vi "FBKdisplay.vi"() -> ()   [LabVIEW 2017]
uses:
  <vilib>/picture/3D Picture Control/NI_3D Picture Control.lvlib
  <vilib>/Utility/miscctls.llb/LVRectTypeDef.ctl
  <vilib>/picture/3D Picture Control/Object/Create Object (name).vi
panel:
  out "x-y":dbl
  out "ForceControl":bool
  out "HorizontalVisualFBK":bool
  out "InvertVisualFbk":bool
  in  "Render Dest":enum16{"Scene Window", "Scene Display"}(ring)
  in  "stop":bool
  in  "Camera Controller":enum16{"None", "Spherical", "Flying"}(ring)=enum."Spherical"
  out "error out":errorcluster
  out "Scene Display":refnum<vi>(3d-picture)
  out "error out 2":errorcluster
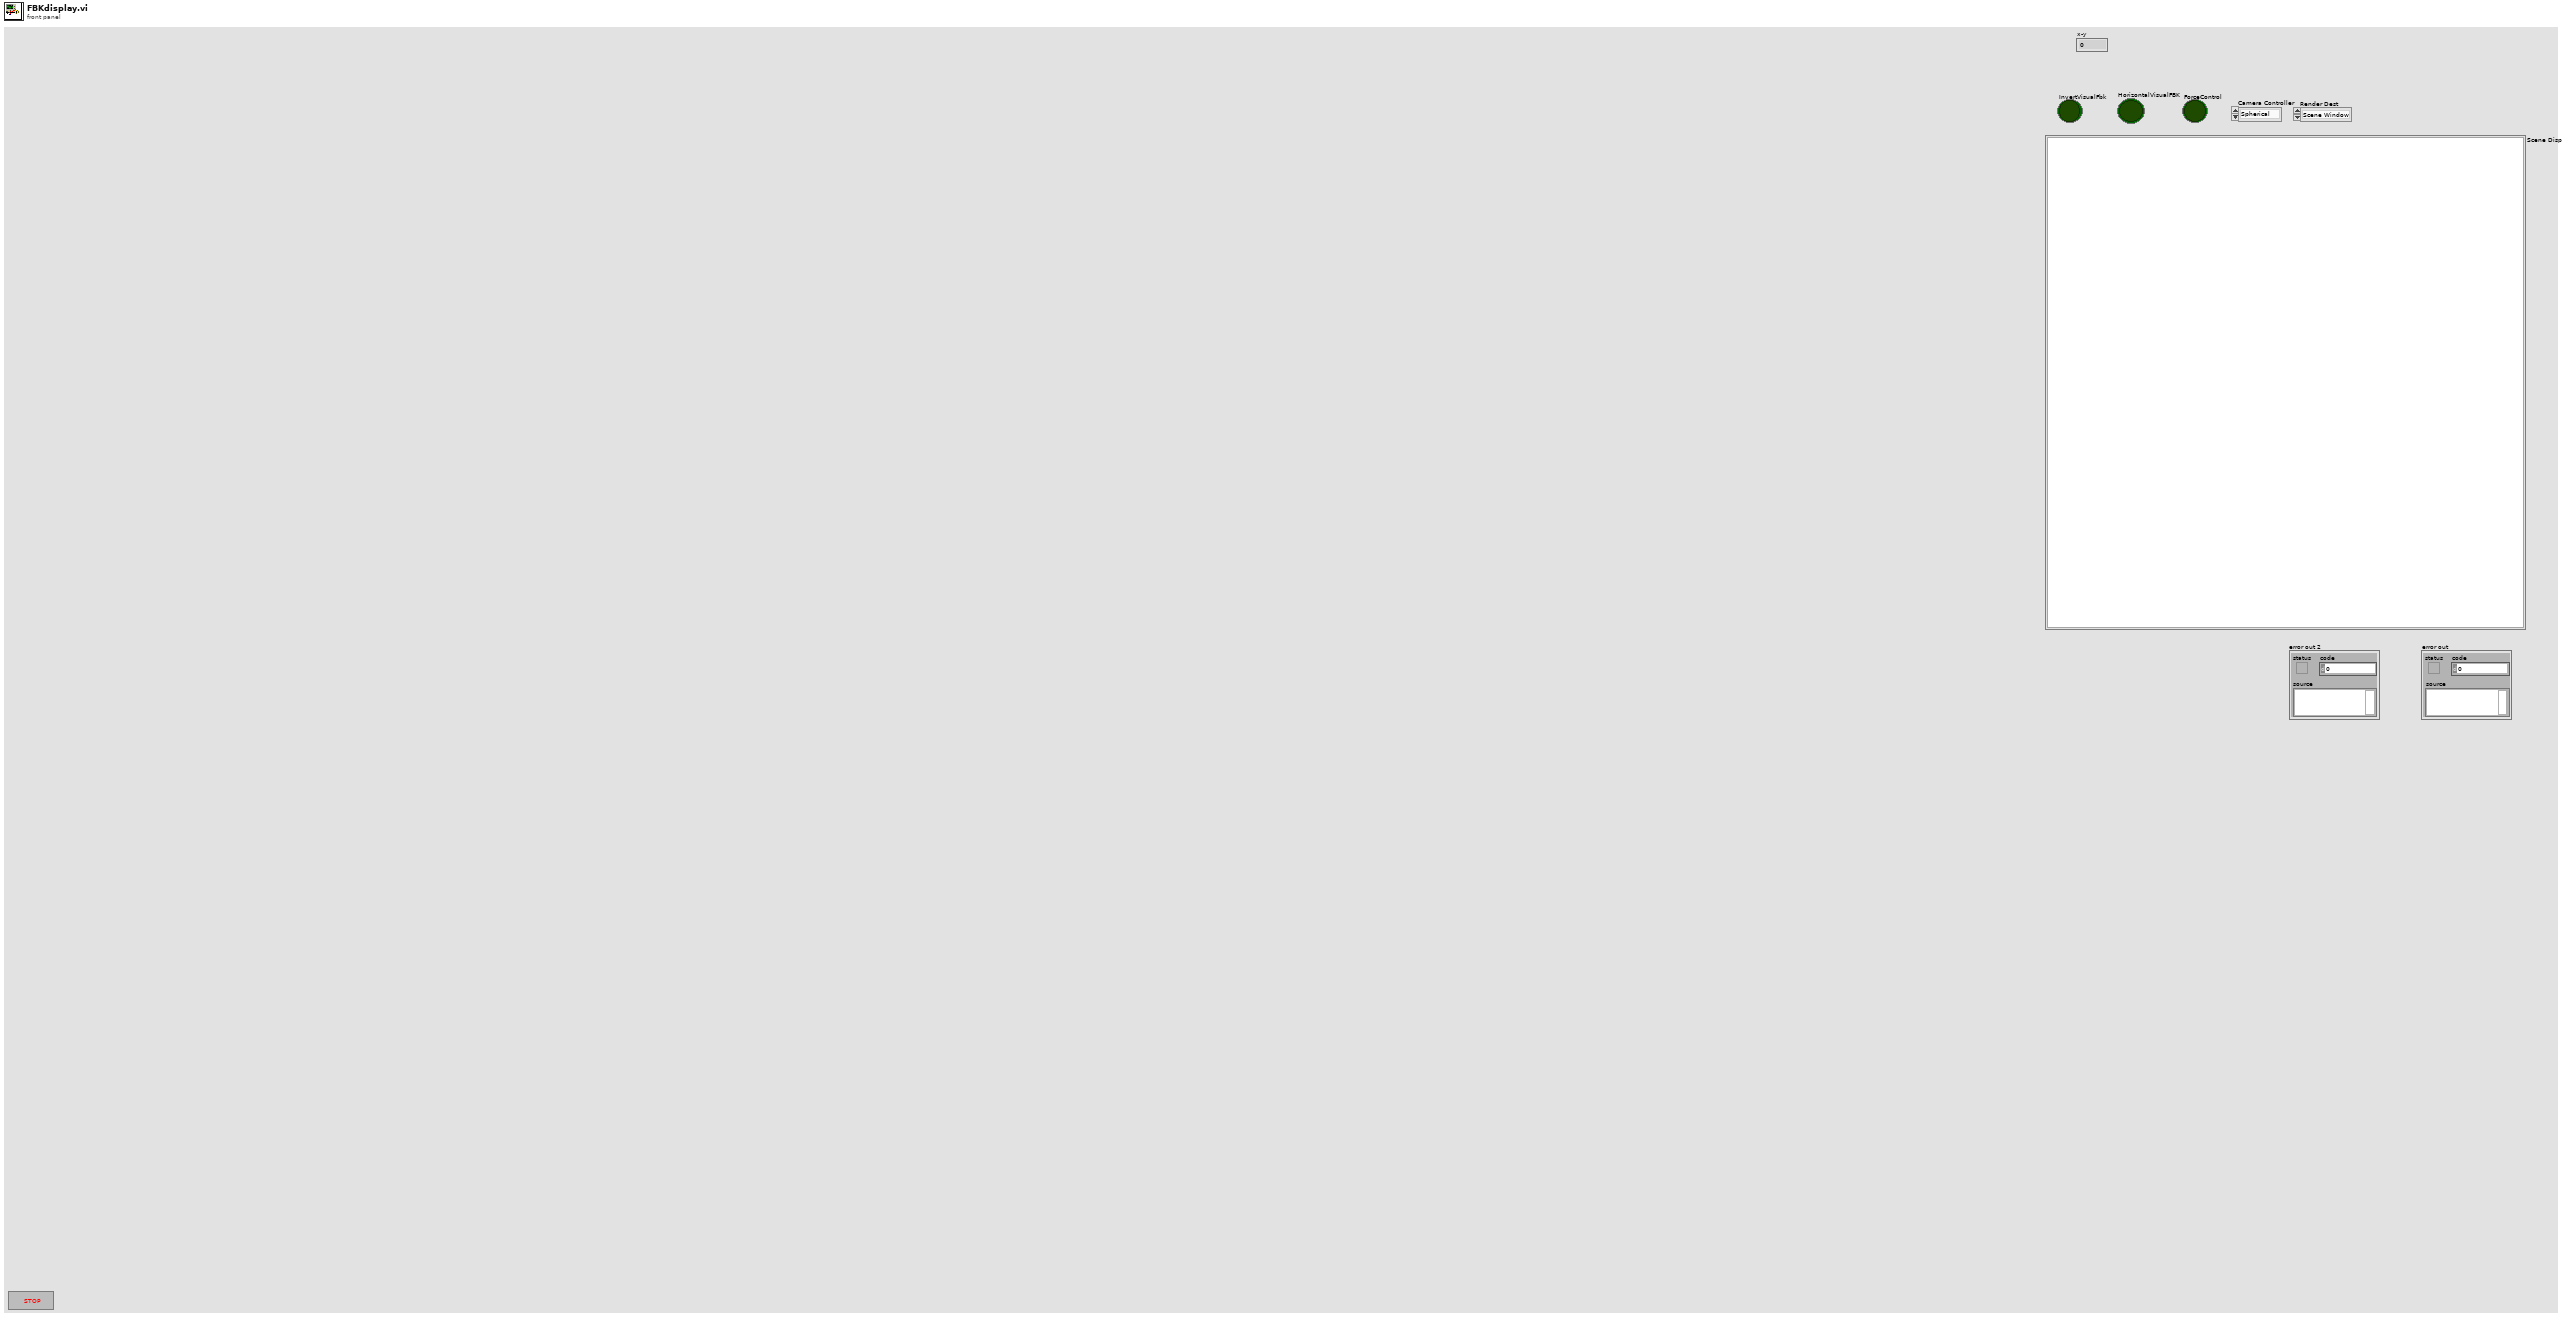
[diagram p1: front panel]
types:
  T1 = enum16{"As a Decal", "With Modulation", "With Blending", "As a replacement"}
  T2 = typedef "LVRectTypeDef.ctl" = cluster{"Left":i16, "Top":i16, "Right":i16, "Bottom":i16}
  T3 = enum16{"Open", "Minimized", "Maximized", "Hidden"}
  T4 = typedef "imagedata.ctl" = cluster{"image type":i32, "image depth":i32, "image":u8[], "mask":u8[], "colors":u32[], "Rectangle":cluster{"left":i16, "top":i16, "right":i16, "bottom":i16}}
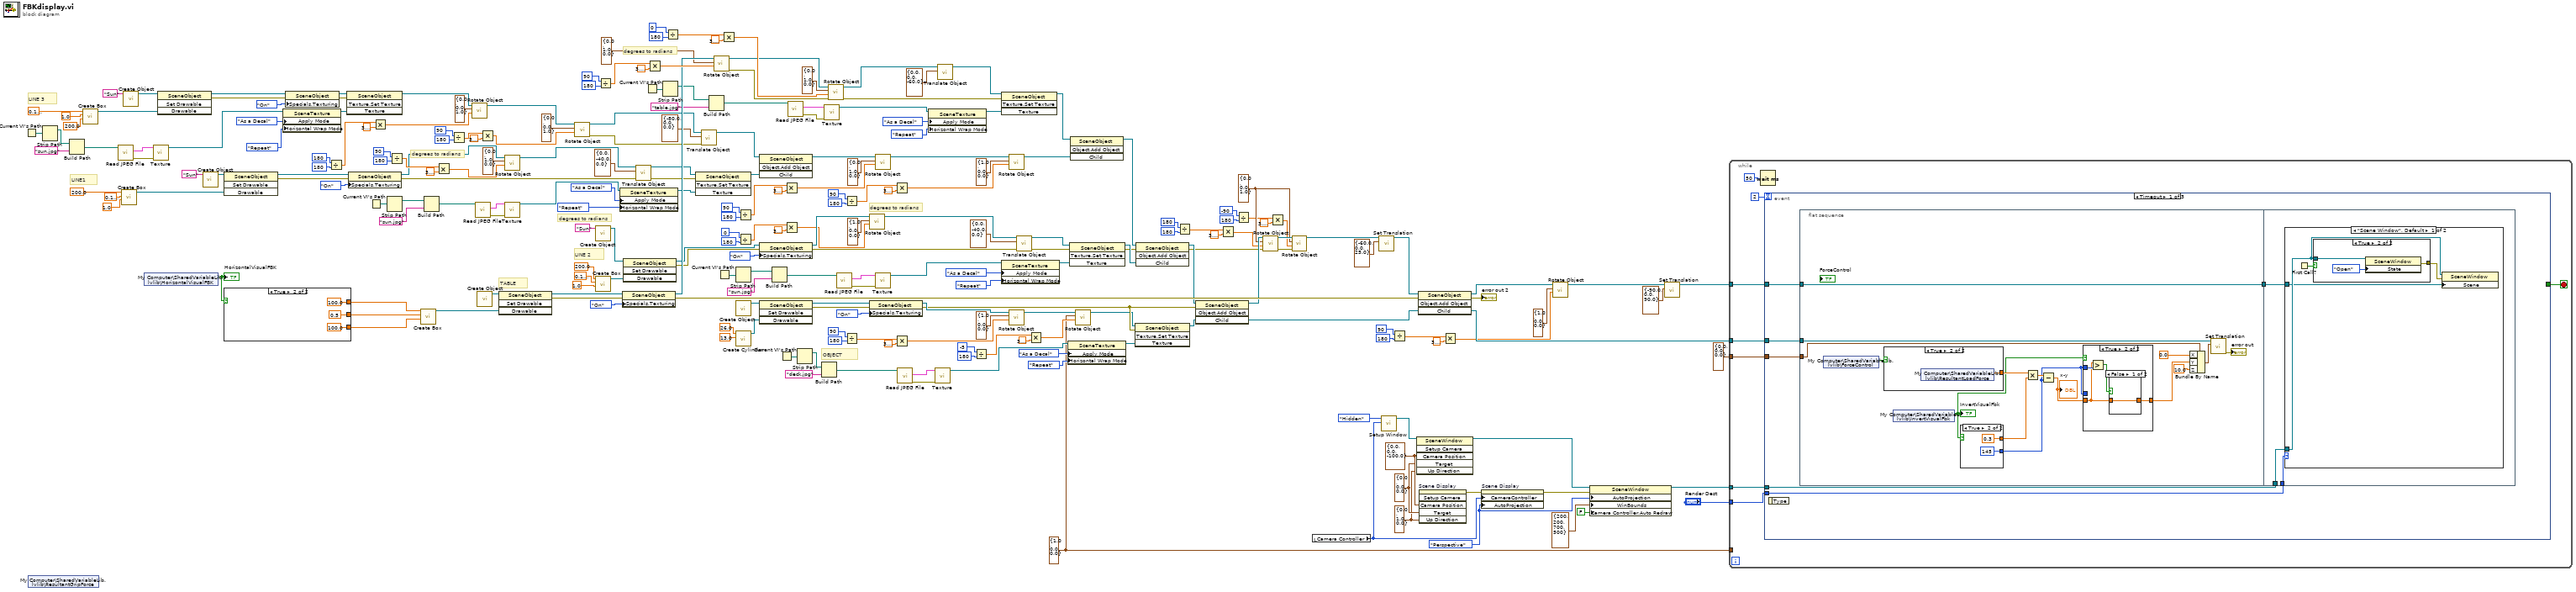
[diagram p0: block diagram]
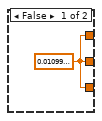
[diagram p2: hidden frame]
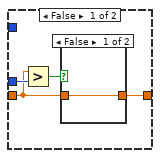
[diagram p3: hidden frame]
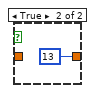
[diagram p4: hidden frame]
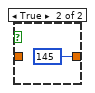
[diagram p5: hidden frame]
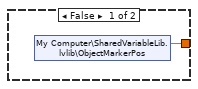
[diagram p6: hidden frame]
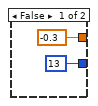
[diagram p7: hidden frame]
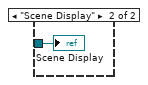
[diagram p9: hidden frame]
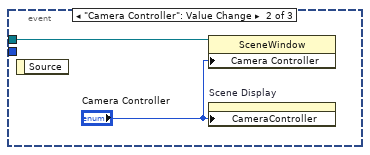
[diagram p10: hidden frame]
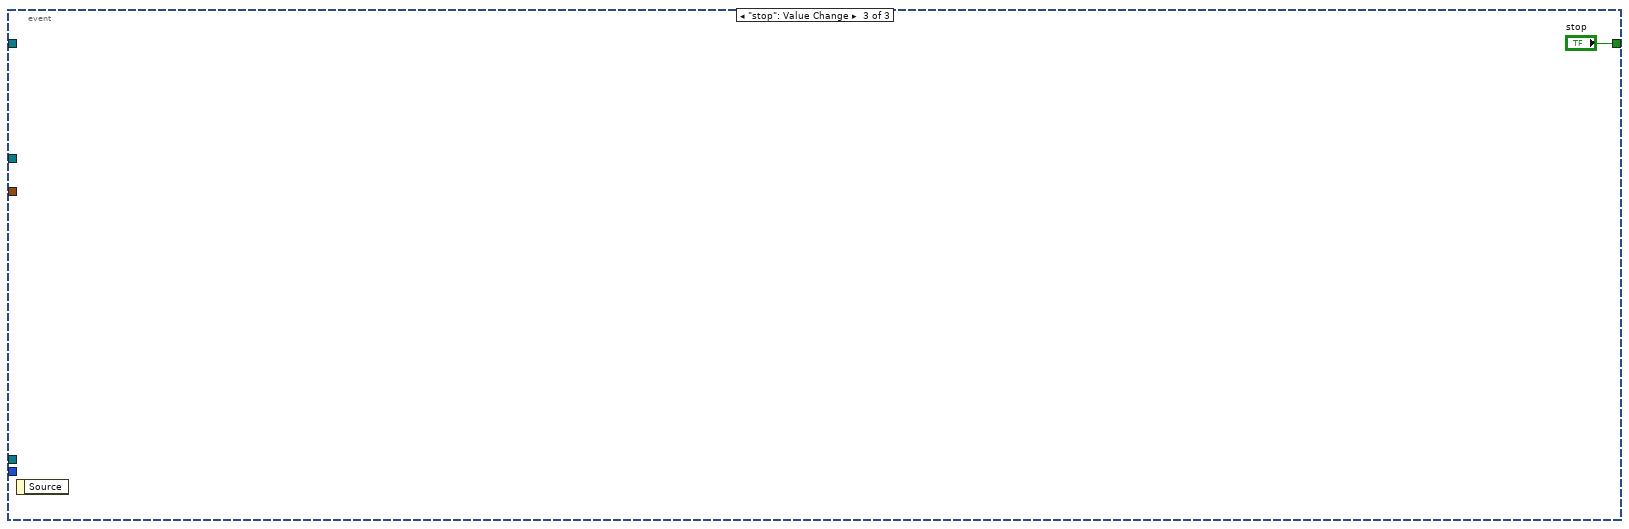
[diagram p11: hidden frame]
diagram:
  w74 = cluster{"X":sgl, "Y":sgl, "Z":sgl} {"X"=0.0, "Y"=0.0, "Z"=1.0} ("Axis")
  w119 = cluster{"X":sgl, "Y":sgl, "Z":sgl} {"X"=1.0, "Y"=0.0, "Z"=0.0} ("Axis")
  w212 = enum16{"None", "Perspective", "Orthographic"}."Perspective" ("Auto Projection Mode")
  w215 = cluster{"X":sgl, "Y":sgl, "Z":sgl} {"X"=0.0, "Y"=1.0, "Z"=0.0} ("Up Direction")
  w216 = cluster{"X":sgl, "Y":sgl, "Z":sgl} {"X"=0.0, "Y"=0.0, "Z"=0.0} ("Target")
  w217 = cluster{"X":sgl, "Y":sgl, "Z":sgl} {"X"=0.0, "Y"=0.0, "Z"=-100.0} ("Camera Position")
  # "degrees to radians"
  # "LINE 3"
  # "OBJECT"
  # "LINE 2"
  # "LINE1"
  # "TABLE"
  # "degrees to radians"
  # "degrees to radians"
  # "degrees to radians"
  n1 = Current VI's Path() -> (path=w110:path)
  n2 = shared-variable "My Computer\\SharedVariableLib.lvlib\\ResultantGripForce"() -> ()  [unwired: 1 in, 2 out]
  n3 = Strip Path(path=w110) -> (stripped path=w109:path)  [unwired: 1 out]
  n4 = Build Path(base path=w109, name or relative path="sun.jpg" ("Name")) -> (appended path=w107:path)
  n5 = call <vilib>:"Create Box.vi"("Length Z"=sgl 200.0 ("Detail"), "Length Y"=sgl 1.0 ("Detail"), "Length X"=sgl 0.1 ("Radius")) -> ("New Box Refnum"=w116:refnum<vi>)  [unwired: 7 in, 1 out]
  n6 = call <vilib>:"Read JPEG File.vi"("path to JPEG file"=w107) -> ("error out"=w111:errorcluster, "image data"=w112:T4)  [unwired: 1 in, 8 out]
  n7 = call <vilib>:"Create Box.vi"("Length Z"=sgl 1.0 ("Detail"), "Length Y"=sgl 0.1 ("Detail"), "Length X"=sgl 200.0 ("Radius")) -> ("New Box Refnum"=w179:refnum<vi>)  [unwired: 7 in, 1 out]
  n8 = call-poly <vilib>:"Create Object.vi"("Name"="Sun") -> ("Scene:New Object"=w117:refnum<vi>)  [unwired: 9 in, 1 out]
  n9 = shared-variable "My Computer\\SharedVariableLib.lvlib\\HorizontalVisualFBK"() -> (w4:bool)  [unwired: 1 in, 1 out]
  "HorizontalVisualFBK" <- w4
  n10 = call <vilib>:"Texture.vi"("error in (no error)"=w111, "Image"=w112) -> ("New Texture Refnum"=w102:refnum<vi>)  [unwired: 9 out]
  n11 = invoke class="SceneObject" method="Set Drawable"(reference=w117, "Drawable"=w116) -> (reference out=w106:refnum<vi>, error out=w105:errorcluster)  [unwired: 2 in, 2 out]
  n12 = call-poly <vilib>:"Create Object.vi"("Name"="Sun") -> ("Scene:New Object"=w180:refnum<vi>)  [unwired: 9 in, 1 out]
  n13 = invoke class="SceneObject" method="Set Drawable"(reference=w180, "Drawable"=w179) -> (reference out=w177:refnum<vi>, error out=w176:errorcluster)  [unwired: 2 in, 2 out]
  n14 = case shown="True" w4 {
    tunnel: [w242 sgl 100.0 ("Radius")] -> w1
    tunnel: [w242 sgl 0.5 ("Radius")] -> w2
    tunnel: [w242 sgl 100.0 ("Radius")] -> w3
    frame False {
      w242 = sgl 0.011 ("Radius")
    }
    frame True {
    }
  }
  n15 = property class="SceneTexture"(reference=w102, "Apply Mode"=T1."As a Decal", "Horizontal Wrap Mode"=enum16{"Clamp", "Repeat"}."Repeat") -> (reference out=w100:refnum<vi>)  [unwired: 1 in, 1 out]
  n16 = property class="SceneObject"(reference=w106, error in=w105, "Specials.Texturing"=enum16{"Inherit Value", "Off", "On"}."On" ("Specials:Texturing")) -> (reference out=w11:refnum<vi>, error out=w10:errorcluster)
  n17 = Divide(x=180, y=180) -> (x/y=w39:dbl)
  n18 = invoke class="SceneObject" method="Texture.Set Texture"(reference=w11, error in=w10, "Texture"=w100) -> (reference out=w44:refnum<vi>)  [unwired: 1 in, 3 out]
  n19 = property class="SceneObject"(reference=w177, error in=w176, "Specials.Texturing"=enum16{"Inherit Value", "Off", "On"}."On" ("Specials:Texturing")) -> (reference out=w159:refnum<vi>, error out=w129:errorcluster)
  n20 = Current VI's Path() -> (path=w169:path)
  n21 = Multiply(x=w39, y=3.141592653589793) -> (x*y=w38:dbl)
  n22 = Strip Path(path=w169) -> (stripped path=w168:path)  [unwired: 1 out]
  n23 = Divide(x=90, y=180) -> (x/y=w160:dbl)
  n24 = call <vilib>:"Create Box.vi"("Length Z"=w1, "Length Y"=w2, "Length X"=w3) -> ("New Box Refnum"=w221:refnum<vi>)  [unwired: 7 in, 1 out]
  n25 = Build Path(base path=w168, name or relative path="sun.jpg" ("Name")) -> (appended path=w166:path)
  n26 = Multiply(x=w160, y=3.141592653589793) -> (x*y=w61:dbl)
  n27 = Divide(x=90, y=180) -> (x/y=w32:dbl)
  n28 = call <vilib>:"Rotate Object.vi"("Angle"=w38, "Axis"=cluster{"X":sgl, "Y":sgl, "Z":sgl} {"X"=0.0, "Y"=0.0, "Z"=1.0}, "Scene.Object In"=w44) -> ("Scene.Object Out"=w36:refnum<vi>)  [unwired: 1 in, 7 out]
  n29 = call <vilib>:"Read JPEG File.vi"("path to JPEG file"=w166) -> ("error out"=w171:errorcluster, "image data"=w172:T4)  [unwired: 1 in, 8 out]
  n30 = call-poly <vilib>:"Create Object.vi"() -> ("Scene:New Object"=w229:refnum<vi>)  [unwired: 10 in, 1 out]
  n31 = Multiply(x=w32, y=3.141592653589793) -> (x*y=w31:dbl)
  n32 = invoke class="SceneObject" method="Set Drawable"(reference=w229, "Drawable"=w221) -> (reference out=w241:refnum<vi>, error out=w240:errorcluster)  [unwired: 2 in, 2 out]
  n33 = call <vilib>:"Texture.vi"("error in (no error)"=w171, "Image"=w172) -> ("New Texture Refnum"=w170:refnum<vi>)  [unwired: 9 out]
  n34 = call <vilib>:"Rotate Object.vi"("Angle"=w61, "Axis"=cluster{"X":sgl, "Y":sgl, "Z":sgl} {"X"=0.0, "Y"=1.0, "Z"=0.0}, "Scene.Object In"=w159) -> ("Scene.Object Out"=w45:refnum<vi>)  [unwired: 1 in, 7 out]
  n35 = call <vilib>:"Rotate Object.vi"("Angle"=w31, "Axis"=cluster{"X":sgl, "Y":sgl, "Z":sgl} {"X"=0.0, "Y"=0.0, "Z"=1.0}, "Scene.Object In"=w36) -> ("error out"=w28:errorcluster, "Scene.Object Out"=w29:refnum<vi>)  [unwired: 1 in, 6 out]
  n36 = call-poly <vilib>:"Create Object.vi"("Name"="Sun") -> ("Scene:New Object"=w157:refnum<vi>)  [unwired: 9 in, 1 out]
  n37 = call <vilib>:"Create Box.vi"("Length Z"=sgl 1.0 ("Detail"), "Length Y"=sgl 0.1 ("Detail"), "Length X"=sgl 200.0 ("Radius")) -> ("New Box Refnum"=w156:refnum<vi>)  [unwired: 7 in, 1 out]
  n38 = Divide(x=90, y=180) -> (x/y=w235:dbl)
  n39 = property class="SceneTexture"(reference=w170, "Apply Mode"=T1."As a Decal", "Horizontal Wrap Mode"=enum16{"Clamp", "Repeat"}."Repeat") -> (reference out=w99:refnum<vi>)  [unwired: 1 in, 1 out]
  n40 = property class="SceneObject"(reference=w241, error in=w240, "Specials.Texturing"=enum16{"Inherit Value", "Off", "On"}."On" ("Specials:Texturing")) -> (reference out=w225:refnum<vi>, error out=w134:errorcluster)
  n41 = invoke class="SceneObject" method="Set Drawable"(reference=w157, "Drawable"=w156) -> (reference out=w154:refnum<vi>, error out=w153:errorcluster)  [unwired: 2 in, 2 out]
  n42 = call <vilib>:"Translate Object.vi"("error in (no error)"=w129, "Translation"=cluster{"X":sgl, "Y":sgl, "Z":sgl} {"X"=0.0, "Y"=-40.0, "Z"=0.0} ("Axis"), "Scene.Object In"=w45) -> ("error out"=w97:errorcluster, "Scene.Object Out"=w98:refnum<vi>)  [unwired: 7 in]
  n43 = Current VI's Path() -> (path=w194:path)
  n44 = Multiply(x=w235, y=3.141592653589793) -> (x*y=w227:dbl)
  n45 = Strip Path(path=w194) -> (stripped path=w193:path)  [unwired: 1 out]
  n46 = Divide(x=0, y=180) -> (x/y=w200:dbl)
  n47 = invoke class="SceneObject" method="Texture.Set Texture"(reference=w98, error in=w97, "Texture"=w99) -> (reference out=w96:refnum<vi>)  [unwired: 1 in, 3 out]
  n48 = call <vilib>:"Translate Object.vi"("error in (no error)"=w28, "Translation"=cluster{"X":sgl, "Y":sgl, "Z":sgl} {"X"=-80.0, "Y"=0.0, "Z"=0.0} ("Axis"), "Scene.Object In"=w29) -> ("Scene.Object Out"=w27:refnum<vi>)  [unwired: 7 in, 1 out]
  n49 = Build Path(base path=w193, name or relative path="table.jpg" ("Name")) -> (appended path=w191:path)
  n50 = call <vilib>:"Rotate Object.vi"("Angle"=w227, "Axis"=cluster{"X":sgl, "Y":sgl, "Z":sgl} {"X"=0.0, "Y"=1.0, "Z"=0.0}, "Scene.Object In"=w225) -> ("error out"=w198:errorcluster, "Scene.Object Out"=w197:refnum<vi>)  [unwired: 1 in, 6 out]
  n51 = Current VI's Path() -> (path=w146:path)
  n52 = Multiply(x=w200, y=3.141592653589793) -> (x*y=w199:dbl)
  n53 = Strip Path(path=w146) -> (stripped path=w145:path)  [unwired: 1 out]
  n54 = call-poly <vilib>:"Create Object.vi"() -> ("Scene:New Object"=w228:refnum<vi>)  [unwired: 10 in, 1 out]
  n55 = call <vilib>:"Create Cylinder.vi"("Radius"=sgl 13.0 ("Detail"), "Height"=sgl 26.0 ("Radius")) -> ("New Cylinder Refnum"=w220:refnum<vi>)  [unwired: 8 in, 1 out]
  n56 = Divide(x=90, y=180) -> (x/y=w65:dbl)
  n57 = Divide(x=0, y=180) -> (x/y=w137:dbl)
  n58 = invoke class="SceneObject" method="Object.Add Object"(reference=w27, "Child"=w96) -> (reference out=w48:refnum<vi>)  [unwired: 2 in, 3 out]
  n59 = property class="SceneObject"(reference=w154, error in=w153, "Specials.Texturing"=enum16{"Inherit Value", "Off", "On"}."On" ("Specials:Texturing")) -> (reference out=w136:refnum<vi>, error out=w93:errorcluster)
  n60 = invoke class="SceneObject" method="Set Drawable"(reference=w228, "Drawable"=w220) -> (reference out=w231:refnum<vi>, error out=w233:errorcluster)  [unwired: 2 in, 2 out]
  n61 = Build Path(base path=w145, name or relative path="sun.jpg" ("Name")) -> (appended path=w143:path)
  n62 = Current VI's Path() -> (path=w187:path)
  n63 = Multiply(x=w65, y=3.141592653589793) -> (x*y=w63:dbl)
  n64 = Multiply(x=w137, y=3.141592653589793) -> (x*y=w59:dbl)
  n65 = call <vilib>:"Read JPEG File.vi"("path to JPEG file"=w191) -> ("error out"=w195:errorcluster, "image data"=w196:T4)  [unwired: 1 in, 8 out]
  n66 = Strip Path(path=w187) -> (stripped path=w186:path)  [unwired: 1 out]
  n67 = Build Path(base path=w186, name or relative path="deck.jpg" ("Name")) -> (appended path=w184:path)
  n68 = call <vilib>:"Texture.vi"("error in (no error)"=w195, "Image"=w196) -> ("New Texture Refnum"=w88:refnum<vi>)  [unwired: 9 out]
  n69 = call <vilib>:"Rotate Object.vi"("error in (no error)"=w198, "Angle"=w199, "Axis"=cluster{"X":sgl, "Y":sgl, "Z":sgl} {"X"=0.0, "Y"=1.0, "Z"=0.0}, "Scene.Object In"=w197) -> ("error out"=w9:errorcluster, "Scene.Object Out"=w7:refnum<vi>)  [unwired: 6 out]
  n70 = call <vilib>:"Read JPEG File.vi"("path to JPEG file"=w143) -> ("error out"=w148:errorcluster, "image data"=w149:T4)  [unwired: 1 in, 8 out]
  n71 = Divide(x=90, y=180) -> (x/y=w55:dbl)
  n72 = Divide(x=90, y=180) -> (x/y=w128:dbl)
  n73 = call <vilib>:"Rotate Object.vi"("Angle"=w59, "Axis"=cluster{"X":sgl, "Y":sgl, "Z":sgl} {"X"=1.0, "Y"=0.0, "Z"=0.0}, "Scene.Object In"=w136) -> ("Scene.Object Out"=w49:refnum<vi>)  [unwired: 1 in, 7 out]
  n74 = property class="SceneObject"(reference=w231, error in=w233, "Specials.Texturing"=enum16{"Inherit Value", "Off", "On"}."On" ("Specials:Texturing")) -> (reference out=w121:refnum<vi>, error out=w15:errorcluster)
  n75 = call <vilib>:"Texture.vi"("error in (no error)"=w148, "Image"=w149) -> ("New Texture Refnum"=w147:refnum<vi>)  [unwired: 9 out]
  n76 = call <vilib>:"Rotate Object.vi"("Angle"=w63, "Axis"=cluster{"X":sgl, "Y":sgl, "Z":sgl} {"X"=0.0, "Y"=1.0, "Z"=0.0}, "Scene.Object In"=w48) -> ("Scene.Object Out"=w52:refnum<vi>)  [unwired: 1 in, 7 out]
  n77 = Multiply(x=w55, y=3.141592653589793) -> (x*y=w54:dbl)
  n78 = Multiply(x=w128, y=3.141592653589793) -> (x*y=w222:dbl)
  n79 = call <vilib>:"Read JPEG File.vi"("path to JPEG file"=w184) -> ("error out"=w189:errorcluster, "image data"=w190:T4)  [unwired: 1 in, 8 out]
  n80 = property class="SceneTexture"(reference=w88, "Apply Mode"=T1."As a Decal", "Horizontal Wrap Mode"=enum16{"Clamp", "Repeat"}."Repeat") -> (reference out=w87:refnum<vi>)  [unwired: 1 in, 1 out]
  n81 = call <vilib>:"Texture.vi"("error in (no error)"=w189, "Image"=w190) -> ("New Texture Refnum"=w188:refnum<vi>)  [unwired: 9 out]
  n82 = call <vilib>:"Translate Object.vi"("Translation"=cluster{"X":sgl, "Y":sgl, "Z":sgl} {"X"=0.0, "Y"=0.0, "Z"=-60.0}, "Scene.Object In"=w7) -> ("Scene.Object Out"=w6:refnum<vi>)  [unwired: 8 in, 1 out]
  n83 = Divide(x=-5, y=180) -> (x/y=w123:dbl)
  n84 = property class="SceneTexture"(reference=w147, "Apply Mode"=T1."As a Decal", "Horizontal Wrap Mode"=enum16{"Clamp", "Repeat"}."Repeat") -> (reference out=w92:refnum<vi>)  [unwired: 1 in, 1 out]
  n85 = invoke class="SceneObject" method="Texture.Set Texture"(reference=w6, error in=w9, "Texture"=w87) -> (reference out=w84:refnum<vi>)  [unwired: 1 in, 3 out]
  n86 = call <vilib>:"Rotate Object.vi"("Angle"=w54, "Axis"=cluster{"X":sgl, "Y":sgl, "Z":sgl} {"X"=1.0, "Y"=0.0, "Z"=0.0}, "Scene.Object In"=w52) -> ("Scene.Object Out"=w51:refnum<vi>)  [unwired: 1 in, 7 out]
  n87 = call <vilib>:"Rotate Object.vi"("Angle"=w222, "Axis"=cluster{"X":sgl, "Y":sgl, "Z":sgl} {"X"=1.0, "Y"=0.0, "Z"=0.0}, "Scene.Object In"=w121) -> ("Scene.Object Out"=w120:refnum<vi>)  [unwired: 1 in, 7 out]
  n88 = call <vilib>:"Translate Object.vi"("error in (no error)"=w93, "Translation"=cluster{"X":sgl, "Y":sgl, "Z":sgl} {"X"=0.0, "Y"=-40.0, "Z"=0.0} ("Axis"), "Scene.Object In"=w49) -> ("error out"=w94:errorcluster, "Scene.Object Out"=w95:refnum<vi>)  [unwired: 7 in]
  n89 = Multiply(x=w123, y=3.141592653589793) -> (x*y=w125:dbl)
  n90 = property class="SceneTexture"(reference=w188, "Apply Mode"=T1."As a Decal", "Horizontal Wrap Mode"=enum16{"Clamp", "Repeat"}."Repeat") -> (reference out=w133:refnum<vi>)  [unwired: 1 in, 1 out]
  n91 = invoke class="SceneObject" method="Texture.Set Texture"(reference=w95, error in=w94, "Texture"=w92) -> (reference out=w91:refnum<vi>, error out=w14:errorcluster)  [unwired: 1 in, 2 out]
  n92 = invoke class="SceneObject" method="Object.Add Object"(reference=w84, "Child"=w51) -> (reference out=w47:refnum<vi>)  [unwired: 2 in, 3 out]
  n93 = call <vilib>:"Rotate Object.vi"("Angle"=w125, "Axis"=w119, "Scene.Object In"=w120) -> ("Scene.Object Out"=w8:refnum<vi>)  [unwired: 1 in, 7 out]
  n94 = invoke class="SceneObject" method="Texture.Set Texture"(reference=w8, error in=w15, "Texture"=w133) -> (reference out=w132:refnum<vi>)  [unwired: 1 in, 3 out]
  n95 = invoke class="SceneObject" method="Object.Add Object"(reference=w47, error in=w14, "Child"=w91) -> (reference out=w46:refnum<vi>, error out=w13:errorcluster)  [unwired: 1 in, 2 out]
  n96 = Divide(x=180, y=180) -> (x/y=w80:dbl)
  n97 = invoke class="SceneObject" method="Object.Add Object"(reference=w46, error in=w15, "Child"=w132) -> (reference out=w83:refnum<vi>, "Child"=w26:refnum<vi>)  [unwired: 1 in, 2 out]
  n98 = Multiply(x=w80, y=3.141592653589793) -> (x*y=w78:dbl)
  n99 = Divide(x=-90, y=180) -> (x/y=w71:dbl)
  n100 = call <vilib>:"Rotate Object.vi"("error in (no error)"=w13, "Angle"=w78, "Axis"=w74, "Scene.Object In"=w83) -> ("error out"=w12:errorcluster, "Scene.Object Out"=w75:refnum<vi>)  [unwired: 6 out]
  n101 = Multiply(x=w71, y=3.141592653589793) -> (x*y=w69:dbl)
  n102 = call <vilib>:"Rotate Object.vi"("error in (no error)"=w12, "Angle"=w69, "Axis"=w74, "Scene.Object In"=w75) -> ("Scene.Object Out"=w68:refnum<vi>)  [unwired: 7 out]
  n103 = local read "Camera Controller"() -> (w209:enum16{"None", "Spherical", "Flying"})
  n104 = call <vilib>:"Set Translation.vi"("Translation"=cluster{"X":sgl, "Y":sgl, "Z":sgl} {"X"=-60.0, "Y"=0.0, "Z"=25.0}, "Scene Object"=w68) -> ("Translated Object"=w77:refnum<vi>)  [unwired: 8 in, 1 out]
  n105 = call <vilib>:"Setup Window.vi"("Camera Controller"=w209, "Window State"=T3."Hidden") -> ("New Window Refnum"=w211:refnum<vi>)  [unwired: 1 in, 8 out]
  n106 = Divide(x=90, y=180) -> (x/y=w22:dbl)
  n107 = invoke class="SceneWindow" method="Setup Camera"(reference=w211, "Camera Position"=w217, "Target"=w216, "Up Direction"=w215) -> (reference out=w218:refnum<vi>)  [unwired: 2 in, 5 out]
  n108 = invoke class="SceneObject" method="Object.Add Object"(reference=w77, error in=w134, "Child"=w26) -> (reference out=w18:refnum<vi>, error out=→"error out 2":errorcluster, "Child"=w131:refnum<vi>)  [unwired: 1 in, 1 out]
  n109 = invoke on="Scene Display" class="SceneGraphDisp (strict)" method="Setup Camera"("Camera Position"=w217, "Target"=w216, "Up Direction"=w215) -> (error out=w214:errorcluster)  [unwired: 3 in, 5 out]
  n110 = Multiply(x=w22, y=3.141592653589793) -> (x*y=w20:dbl)
  n111 = property on="Scene Display" class="SceneGraphDisp (strict)"(error in=w214, "CameraController"=w209, "AutoProjection"=w212) -> (error out=w213:errorcluster)  [unwired: 1 in, 1 out]
  n112 = call <vilib>:"Rotate Object.vi"("Angle"=w20, "Axis"=cluster{"X":sgl, "Y":sgl, "Z":sgl} {"X"=1.0, "Y"=0.0, "Z"=0.0}, "Scene.Object In"=w18) -> ("Scene.Object Out"=w17:refnum<vi>)  [unwired: 1 in, 7 out]
  n113 = property class="SceneWindow"(reference=w218, error in=w213, "AutoProjection"=w212, "WinBounds"=T2 {"Left"=200, "Top"=200, "Right"=700, "Bottom"=500} ("Window Bounds"), "Camera Controller.Auto Redraw"=FALSE ("Camera Controller:Auto Redraw")) -> (reference out=w205:refnum<vi>)  [unwired: 1 out]
  n114 = call <vilib>:"Set Translation.vi"("Translation"=cluster{"X":sgl, "Y":sgl, "Z":sgl} {"X"=-90.0, "Y"=0.0, "Z"=90.0}, "Scene Object"=w17) -> ("Translated Object"=w16:refnum<vi>)  [unwired: 8 in, 1 out]
  n115 = while {
    tunnel: w131 -> [w250]
    tunnel: w16 -> [w251]
    tunnel: "Render Dest" -> [w247]
    tunnel: w205 -> [w249]
    tunnel: cluster{"X":sgl, "Y":sgl, "Z":sgl} {"X"=0.0, "Y"=0.0, "Z"=0.0} ("Translation") -> [w246]
    tunnel: w119 -> [_]
    stop <- w248 stop-if-true
    n116 = Wait (ms)(milliseconds to wait=u32 50) -> ()  [unwired: 1 out]
    n117 = event shown="[0] Timeout" {
      selector: _ -> [_ _ _]
      dyn-events: _ -> [_ _ _]
      timeout: 2 -> [_ _ _]
      tunnel: [_ _ "stop"] -> w248
      tunnel: w251 -> [w258 _ _]
      tunnel: w250 -> [w257 _ _]
      tunnel: w246 -> [w256 _ _]
      tunnel: w247 -> [w255 _ _]
      tunnel: w249 -> [w254 w305 _]
      event Timeout {
        n118 = event-data() -> ()  [unwired: 2 out]
        n119 = flat-sequence {
          tunnel: [w274] -> w259
          tunnel: w256 -> [w266]
          tunnel: w257 -> [w267]
          tunnel: w258 -> [w274]
          tunnel: w259 -> [w295]
          tunnel: w255 -> [w294]
          tunnel: w254 -> [w293]
          frame #0 {
            n120 = shared-variable "My Computer\\SharedVariableLib.lvlib\\ForceControl"() -> (w264:bool)  [unwired: 1 in, 1 out]
            n121 = case shown="True" w264 {
              tunnel: [w287 w288] -> w265
              frame False {
                n122 = shared-variable "My Computer\\SharedVariableLib.lvlib\\ObjectMarkerPos"() -> (w287:dbl)  [unwired: 1 in, 1 out]
              }
              frame True {
                n123 = shared-variable "My Computer\\SharedVariableLib.lvlib\\ResultantLoadForce"() -> (w288:dbl)  [unwired: 1 in, 1 out]
              }
            }
            n124 = shared-variable "My Computer\\SharedVariableLib.lvlib\\InvertVisualFbk"() -> (w263:bool)  [unwired: 1 in, 1 out]
            "InvertVisualFbk" <- w263
            n125 = case shown="True" w263 {
              tunnel: [13 145] -> w260
              tunnel: [-0.3 0.3] -> w268
              frame False {
              }
              frame True {
              }
            }
            n126 = Multiply(x=w265, y=w268) -> (x*y=w269:dbl)
            n127 = Subtract(x=w269, y=w260) -> (x-y=w262:dbl)
            "x-y" <- w262
            n128 = case shown="True" w263 {
              tunnel: w262 -> [w275 w281]
              tunnel: w260 -> [w278 _]
              tunnel: [w276 w282] -> w261
              tunnel: w260 -> [_ w283]
              frame False {
                n129 = Greater?(x=w275, y=w278) -> (0:w277:bool)
                n130 = case shown="False" w277 {
                  tunnel: [w279 13] -> w276
                  tunnel: w275 -> [w279 _]
                  frame False {
                  }
                  frame True {
                  }
                }
              }
              frame True {
                n131 = Greater?(x=w281, y=w283) -> (0:w284:bool)
                n132 = case shown="False" w284 {
                  tunnel: [w285 145] -> w282
                  tunnel: w281 -> [w285 _]
                  frame False {
                  }
                  frame True {
                  }
                }
              }
            }
            n133 = Bundle By Name(cluster=w266, "X"=sgl 0.0, "Y"=w261, "Z"=sgl 10.0) -> (w271:cluster{"X":sgl, "Y":sgl, "Z":sgl})
            n134 = call <vilib>:"Set Translation.vi"("Translation"=w271, "Scene Object"=w267) -> ("error out"=→"error out":errorcluster)  [unwired: 8 in, 1 out]
          }
          frame #1 {
            n135 = case shown="\"Scene Window\", Default" w294 {
              tunnel: w293 -> [w297 _]
              tunnel: w295 -> [w296 w303]
              frame "Scene Window", Default {
                n136 = First Call?() -> (First Call?: T/F=w298:bool)
                n137 = case shown="True" w298 {
                  tunnel: w297 -> [_ w302]
                  tunnel: [_ w301] -> w299
                  frame False {
                  }
                  frame True {
                    n138 = property class="SceneWindow"(reference=w302, "State"=T3."Open" ("Window State")) -> (error out=w301:errorcluster)  [unwired: 1 in, 1 out]
                  }
                }
                n139 = property class="SceneWindow"(reference=w297, error in=w299, "Scene"=w296) -> ()  [unwired: 2 out]
              }
              frame "Scene Display" {
                "Scene Display" <- w303
              }
            }
          }
        }
      }
      event "Camera Controller": Value Change {
        n140 = event-data() -> ()  [unwired: 2 out]
        n141 = property class="SceneWindow"(reference=w305, "Camera Controller"="Camera Controller") -> ()  [unwired: 1 in, 2 out]
        n142 = property on="Scene Display" class="SceneGraphDisp (strict)"("CameraController"="Camera Controller") -> ()  [unwired: 2 in, 2 out]
      }
      event "stop": Value Change {
        n143 = event-data() -> ()  [unwired: 2 out]
      }
    }
  }
